vi "test_LoadCommandlineArgs_AddPackedLibWithPath.vi"() -> (3 "Pass?":bool)   [LabVIEW 2019, in "Tests.SolutionBuilder.lvlib"]
uses:
  Tests.SolutionBuilder.lvlib
  SolutionBuilder/Community/Options.ctl
  SolutionBuilder/SolutionBuilder.lvclass
  SolutionBuilder/ProjectItem/ProjectItem.lvclass
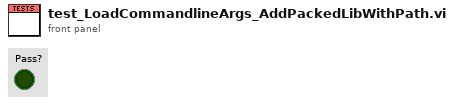
[diagram p1: front panel]
types:
  T1 = typedef "SolutionBuilder.lvlib/SolutionBuilder.lvclass/Options.ctl" = cluster{"Path":path, "Preview?":bool, "Quiet?":bool, "Log file":path, "Success file":path, "Rebuild?":bool, "Keep split projects?":bool}
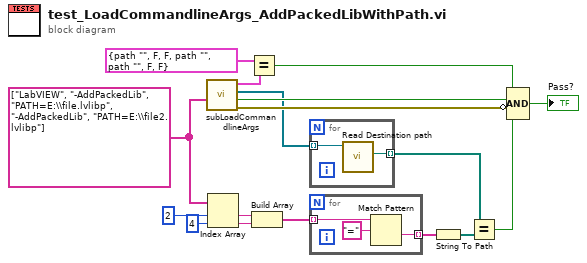
[diagram p0: block diagram]
diagram:
  w10 = string[] ["LabVIEW", "-AddPackedLib", "PATH=E:\\file.lvlibp", "-AddPackedLib", "PATH=E:\\file2.lvlibp"] ("App.Args")
  n1 = call "subLoadCommandlineArgs.vi"("App.Args"=w10) -> ("error out"=w15:errorcluster, "From command line?"=w12:bool, "Pre-built libraries"=w11:refnum<class "ProjectItem.lvclass">[], "Options"=w14:T1)  [unwired: 6 in, 1 out]
  n2 = Index Array(array=w10, index #1=2 ("index"), index #2=4 ("index")) -> (element #1=w7:string, element #2=w6:string)
  n3 = Equal?(x=T1 {"Path"=path "", "Preview?"=FALSE, "Quiet?"=FALSE, "Log file"=path "", "Success file"=path "", "Rebuild?"=FALSE, "Keep split projects?"=FALSE} ("Options"), y=w14) -> (x = y?=w13:bool)
  n4 = Build Array(w7, w6) -> (w2:string[])
  n5 = for {
    tunnel: w11 -> [w19] mode=indexing
    tunnel: [w18] -> w4 mode=indexing
    n6 = call "Read Destination path.vi"("ProjectItem in"=w19) -> ("Destination path"=w18:path)  [unwired: 9 in, 1 out]
  }
  n7 = for {
    tunnel: w2 -> [w22] mode=indexing
    tunnel: [w21] -> w1 mode=indexing
    n8 = Match Pattern(string=w22, regular expression="=") -> (after substring=w21:string)  [unwired: 1 in, 3 out]
  }
  n9 = String To Path(string=w1) -> (path=w5:path[])
  n10 = Equal?(x=w4, y=w5) -> (x = y?=w3:bool)
  n11 = Compound Arithmetic op=AND(w13, w12, invert w15, w3) -> (→"Pass?":bool)
